vi "tabctrl.vi"() -> ()   [LabVIEW 2021]
panel:
  in  "OK 2":bool
  in  "OK":bool
  in  "Tab Control":enum32{"Page 1", "Page 2"}(tab)
  out "Meter":dbl(knob) scale=0.0..10.0
  out "Gauge":dbl(knob) scale=0.0..10.0
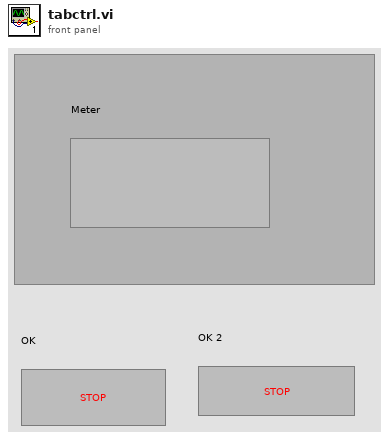
[diagram p1: front panel]
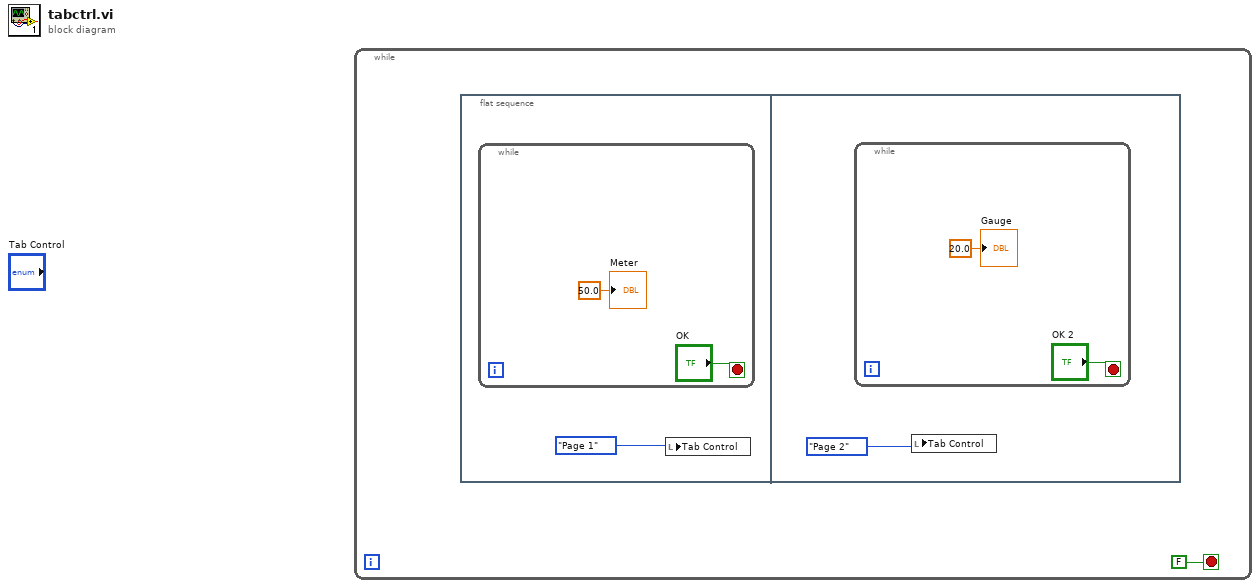
[diagram p0: block diagram]
diagram:
  n1 = while {
    stop <- FALSE stop-if-true
    n2 = flat-sequence {
      frame #0 {
        n3 = while {
          stop <- "OK" stop-if-true
          "Meter" <- 50.0 ("Meter")
        }
        n4 = local write "Tab Control"(enum32{"Page 1", "Page 2"}."Page 1" ("Tab Control")) -> ()
      }
      frame #1 {
        n5 = while {
          stop <- "OK 2" stop-if-true
          "Gauge" <- 20.0 ("Gauge")
        }
        n6 = local write "Tab Control"(enum32{"Page 1", "Page 2"}."Page 2" ("Tab Control")) -> ()
      }
    }
  }
